vi "Spiral.vi"(2 "Loop count":dbl=3.0, 3 "X, Y stride (mm)":dbl[](array[numeric])=[1.0, 1.0], 4 "XY center (mm)":dbl[](array[numeric])) -> (1 "Spiral coordinates":dbl[][](array[numeric]))   [LabVIEW 2018]
uses:
  <vilib>/Utility/file.llb/Write Delimited Spreadsheet (DBL).vi
panel:
  # "Equivalent Python code:\n\ndef spiral(loop):\n    dx, dy = 0, -1\n    bx, by = [0], [0]\n    for i in range((1+2*loop)**2):\n        if bx[i] == by[i] or (bx[i] < 0 and bx[i] == -by[i]) or (bx[i] > 0 and bx[i] == 1-by[i]):\n            dx, dy = -dy, dx\n        if (abs(bx[i]+dx) <= loop) and (abs(by[i]+dy) <= loop):\n            bx.append(bx[i]+dx)\n            by.append(by[i]+dy)\n    return bx, by\n\ntest = np.array(spiral(5))\nplt.plot(Xcenter+scaleX*test[0], Ycenter+scaleY*test[1], '-o')"
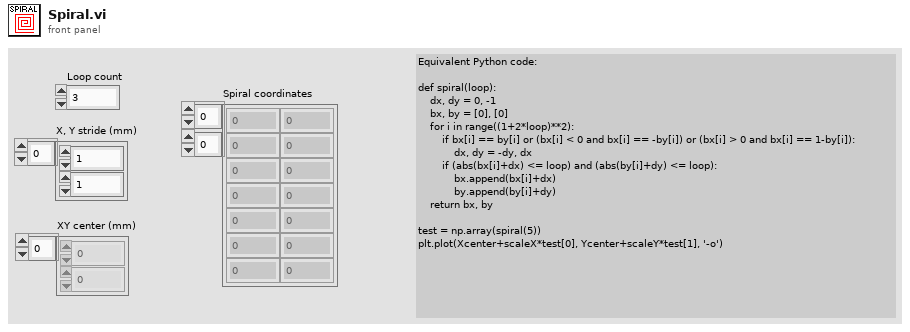
[diagram p1: front panel]
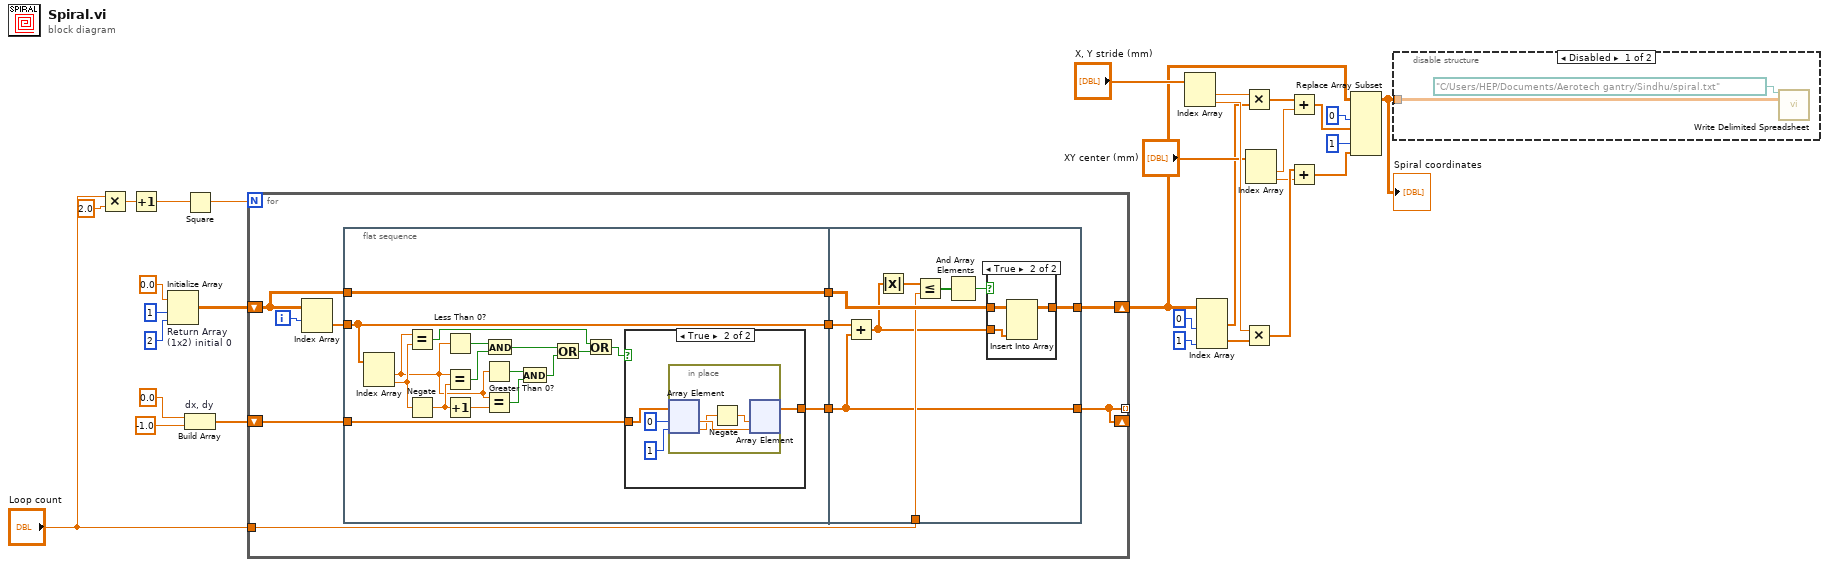
[diagram p0: block diagram]
diagram:
  n1 = Multiply(x="Loop count", y=2.0) -> (x*y=w21:dbl)
  n2 = Increment(x=w21) -> (x+1=w20:dbl)
  n3 = Initialize Array "Return Array\n(1x2) initial 0"(0.0 ("element"), 1 ("dimension size"), 2 ("dimension size")) -> (w29:dbl[][])
  n4 = Square(x=w20) -> (x^2=w24:dbl)
  n5 = Build Array "dx, dy"(0.0 ("element"), -1.0 ("element")) -> (w23:dbl[])
  n6 = for {
    N: w24 -> [_]
    shift-right: [w40] -> w8
    shift-left: w29 -> [w39]
    tunnel: "Loop count" -> [w36]
    tunnel: [w31] -> _ mode=indexing
    shift-right: [w31] -> _
    shift-left: w23 -> [w33]
    i -> [w38]
    n7 = Index Array(array=w39, index (row)=w38) -> (element=w37:dbl[])  [unwired: 1 in]
    n8 = flat-sequence {
      tunnel: w37 -> [w56]
      tunnel: w39 -> [w57]
      tunnel: [w57] -> w35
      tunnel: [w56] -> w34
      tunnel: w33 -> [w47]
      tunnel: [w46] -> w32
      tunnel: [w74] -> w40
      tunnel: w36 -> [w69]
      tunnel: w35 -> [w73]
      tunnel: w34 -> [w72]
      tunnel: w32 -> [w67]
      tunnel: [w67] -> w31
      frame #0 {
        n9 = Index Array(array=w56) -> (element #1=w48:dbl, element #2=w52:dbl)  [unwired: 2 in]
        n10 = Equal?(x=w48, y=w52) -> (x = y?=w41:bool)
        n11 = Negate(x=w52) -> (-x=w49:dbl)
        n12 = Less Than 0?(x=w48) -> (x < 0?=w55:bool)
        n13 = Equal?(x=w48, y=w49) -> (x = y?=w53:bool)
        n14 = Increment(x=w49) -> (x+1=w50:dbl)
        n15 = Greater Than 0?(x=w48) -> (x > 0?=w54:bool)
        n16 = Equal?(x=w48, y=w50) -> (x = y?=w51:bool)
        n17 = And(x=w55, y=w53) -> (x .and. y?=w44:bool)
        n18 = And(x=w54, y=w51) -> (x .and. y?=w45:bool)
        n19 = Or(x=w44, y=w45) -> (x .or. y?=w42:bool)
        n20 = Or(x=w41, y=w42) -> (x .or. y?=w43:bool)
        n21 = case shown="True" w43 {
          tunnel: w47 -> [w58 w59]
          tunnel: [w58 w60] -> w46
          frame False {
          }
          frame True {
            n22 = in-place {
              n23 = in-place-array #1(w59, 0, 1) -> (w65:dbl, w63:dbl)
              n24 = Negate(x=w63) -> (-x=w64:dbl)
              n25 = in-place-array #1(w64, w65) -> (w60:dbl[])  [unwired: 2 out]
            }
          }
        }
      }
      frame #1 {
        n26 = Add(x=w72, y=w67) -> (x+y=w66:dbl[])
        n27 = Absolute Value(x=w66) -> (abs(x)=w70:dbl[])
        n28 = Less Or Equal?(x=w70, y=w69) -> (x <= y?=w68:bool[])
        n29 = And Array Elements(Boolean array=w68) -> (logical AND=w71:bool)
        n30 = case shown="True" w71 {
          tunnel: [w75 w78] -> w74
          tunnel: w73 -> [w75 w77]
          tunnel: w66 -> [_ w76]
          frame False {
          }
          frame True {
            n31 = Insert Into Array(array=w77, new element=w76) -> (w78:dbl[][])  [unwired: 2 in]
          }
        }
      }
    }
  }
  n32 = Index Array(array="X, Y stride (mm)") -> (element #1=w17:dbl, element #2=w16:dbl)  [unwired: 2 in]
  n33 = Index Array(array=w8, index (col) #1=0 ("disabled index (col)"), index (col) #2=1 ("index (col)")) -> (element #1=w5:dbl[], element #2=w3:dbl[])  [unwired: 2 in]
  n34 = Multiply(x=w17, y=w5) -> (x*y=w12:dbl[])
  n35 = Multiply(x=w16, y=w3) -> (x*y=w14:dbl[])
  n36 = Index Array(array="XY center (mm)") -> (element #1=w11:dbl, element #2=w13:dbl)  [unwired: 2 in]
  n37 = Add(x=w12, y=w11) -> (x+y=w4:dbl[])
  n38 = Add(x=w14, y=w13) -> (x+y=w2:dbl[])
  n39 = Replace Array Subset(array=w8, new element #1=w4, index (col) #1=0 ("disabled index (col)"), new element #2=w2, index (col) #2=1 ("index (col)")) -> (w1:dbl[][])  [unwired: 2 in]
  "Spiral coordinates" <- w1
  n40 = disable-structure shown="Disabled" {
    disable-tunnel: w1 -> [w79 _]
    frame Disabled {
      n41 = call-poly <vilib>:"Write Delimited Spreadsheet.vi"("file path (dialog if empty)"=path "C:/Users/HEP/Documents/Aerotech gantry/Sindhu/spiral.txt", "2D data"=w79) -> ()  [unwired: 12 in, 2 out]
    }
    frame Enabled {
    }
  }
